vi "draw a line.vi"(8 "y1":dbl, 9 "y0":dbl, 10 "x1":dbl, 11 "x0":dbl) -> (3 "output cluster":cluster{dbl[], dbl[]})   [LabVIEW 2015]
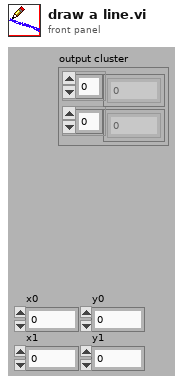
[diagram p1: front panel]
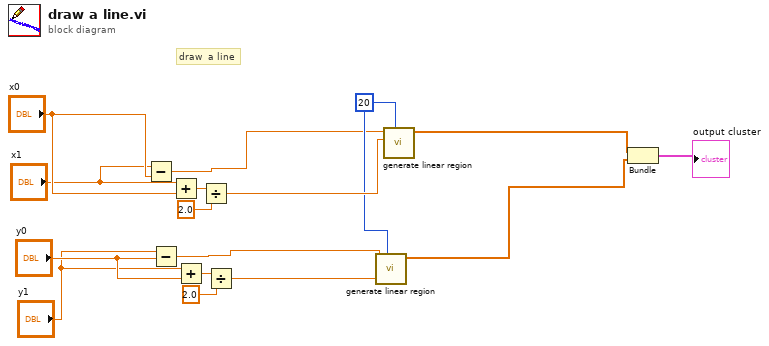
[diagram p0: block diagram]
diagram:
  w8 = 20 ("number of  grid points")
  # "draw  a line"
  n1 = Subtract(x="x1", y="x0") -> (x-y=w2:dbl)
  n2 = Subtract(x="y1", y="y0") -> (x-y=w1:dbl)
  n3 = Add(x="x1", y="x0") -> (x+y=w15:dbl)
  n4 = Add(x="y1", y="y0") -> (x+y=w13:dbl)
  n5 = Divide(x=w15, y=2.0) -> (x/y=w9:dbl)
  n6 = Divide(x=w13, y=2.0) -> (x/y=w5:dbl)
  n7 = call "generate linear region.vi"("number of  grid points"=w8, "center"=w5, "delta"=w1) -> ("real axis"=w4:dbl[])  [unwired: 8 in]
  n8 = call "generate linear region.vi"("number of  grid points"=w8, "center"=w9, "delta"=w2) -> ("real axis"=w16:dbl[])  [unwired: 8 in]
  n9 = Bundle("real axis"=w16, "real axis"=w4) -> (→"output cluster":cluster{"real axis":dbl[], "real axis":dbl[]})  [unwired: 1 in]
